vi "RobotDrive-HaloCalc.vi"(1 "QwikTurnButton":bool, 5 "Left axis value":dbl, 9 "Right axis value":dbl, 12 "Sensitivity":dbl, 13 "QuikTurn Sensitivity":dbl) -> (8 "Left Output":dbl, 10 "Right Output":dbl)   [LabVIEW 2016]
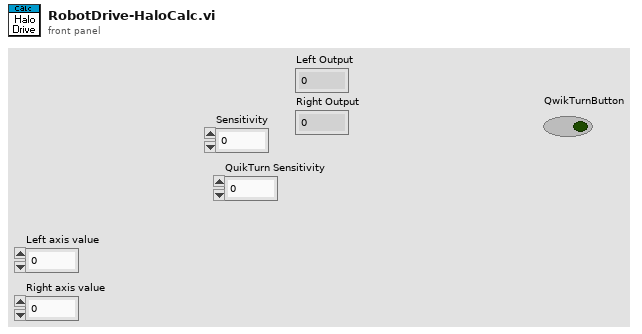
[diagram p1: front panel]
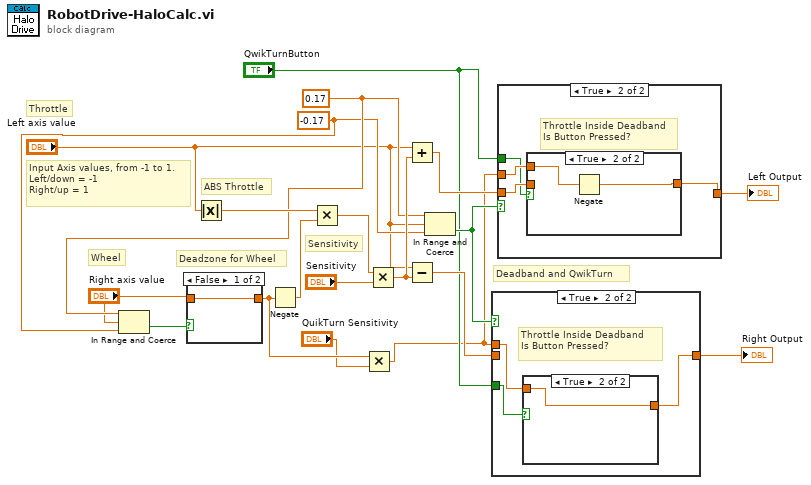
[diagram p0: block diagram]
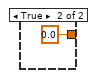
[diagram p2: hidden frame]
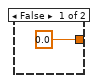
[diagram p5: hidden frame]
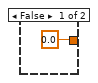
[diagram p8: hidden frame]
diagram:
  w9 = -0.17 ("lower limit")
  w10 = 0.17 ("upper limit")
  # "Deadzone for Wheel"
  # "Deadband and QwikTurn"
  # "Sensitivity"
  # "Wheel"
  # "Throttle"
  # "ABS Throttle"
  # "Input Axis values, from -1 to 1.\nLeft/down = -1\nRight/up = 1"
  n1 = In Range and Coerce(upper limit=w10, x="Right axis value", lower limit=w9) -> (In Range?=w11:bool)  [unwired: 1 out]
  n2 = case shown="False" w11 {
    tunnel: "Right axis value" -> [w20 _]
    tunnel: [w20 0.0 ("Right axis value")] -> w4
    frame False {
    }
    frame True {
    }
  }
  n3 = Absolute Value(x="Left axis value") -> (abs(x)=w19:dbl)
  n4 = Negate(x=w4) -> (-x=w16:dbl)
  n5 = Multiply(x=w19, y=w16) -> (x*y=w18:dbl)
  n6 = Multiply(x=w4, y="QuikTurn Sensitivity") -> (x*y=w3:dbl)
  n7 = Multiply(x=w18, y="Sensitivity") -> (x*y=w17:dbl)
  n8 = Add(x="Left axis value", y=w17) -> (x+y=w12:dbl)
  n9 = Subtract(x="Left axis value", y=w17) -> (x-y=w13:dbl)
  n10 = In Range and Coerce(upper limit=w10, x="Left axis value", lower limit=w9) -> (In Range?=w7:bool)  [unwired: 1 out]
  n11 = case shown="True" w7 {
    tunnel: [w25 w30] -> w14
    tunnel: w13 -> [w24 _]
    tunnel: w3 -> [w23 w29]
    tunnel: "QwikTurnButton" -> [w22 w28]
    frame False {
      # "Throttle Outside Deadband\nIs Button Pressed?"
      n12 = case shown="True" w22 {
        tunnel: w24 -> [w26 w27]
        tunnel: [w26 w27] -> w25
        tunnel: w23 -> [_ _]
        frame False {
        }
        frame True {
        }
      }
    }
    frame True {
      # "Throttle Inside Deadband\nIs Button Pressed?"
      n13 = case shown="True" w28 {
        tunnel: [0.0 w32] -> w30
        tunnel: w29 -> [_ w32]
        frame False {
        }
        frame True {
        }
      }
    }
  }
  "Right Output" <- w14
  n14 = case shown="True" w7 {
    tunnel: w12 -> [w35 w40]
    tunnel: [w36 w41] -> w15
    tunnel: w3 -> [w34 w42]
    tunnel: "QwikTurnButton" -> [w33 w39]
    frame False {
      # "Throttle Outside Deadband\nIs Button Pressed?"
      n15 = case shown="True" w33 {
        tunnel: w35 -> [w37 w38]
        tunnel: [w37 w38] -> w36
        tunnel: w34 -> [_ _]
        frame False {
        }
        frame True {
        }
      }
    }
    frame True {
      # "Throttle Inside Deadband\nIs Button Pressed?"
      n16 = case shown="True" w39 {
        tunnel: w42 -> [_ w45]
        tunnel: [0.0 w44] -> w41
        tunnel: w40 -> [_ _]
        frame False {
        }
        frame True {
          n17 = Negate(x=w45) -> (-x=w44:dbl)
        }
      }
    }
  }
  "Left Output" <- w15
